vi "Configure Module.vi"(8 "error in (no error)":errorcluster, 10 "IOV ref in":refnum<k21>, 11 "9478 in":refnum<class "9478.lvclass">) -> (0 "error out":errorcluster, 2 "IOV ref out":refnum<k21>, 3 "9478 out":refnum<class "9478.lvclass">)   [LabVIEW 2019, in "Modules.lvlib" / "9478.lvclass"]
uses:
  9478.lvclass
  9478.lvclass/9478.ctl
  <resource>/objmgr/cRIO.rc
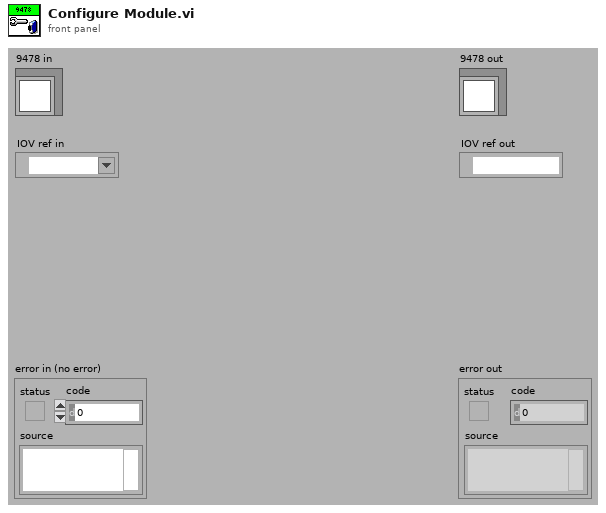
[diagram p1: front panel]
types:
  T1 = typedef "Modules.lvlib/9478.lvclass/Active Limit.ctl" = u8
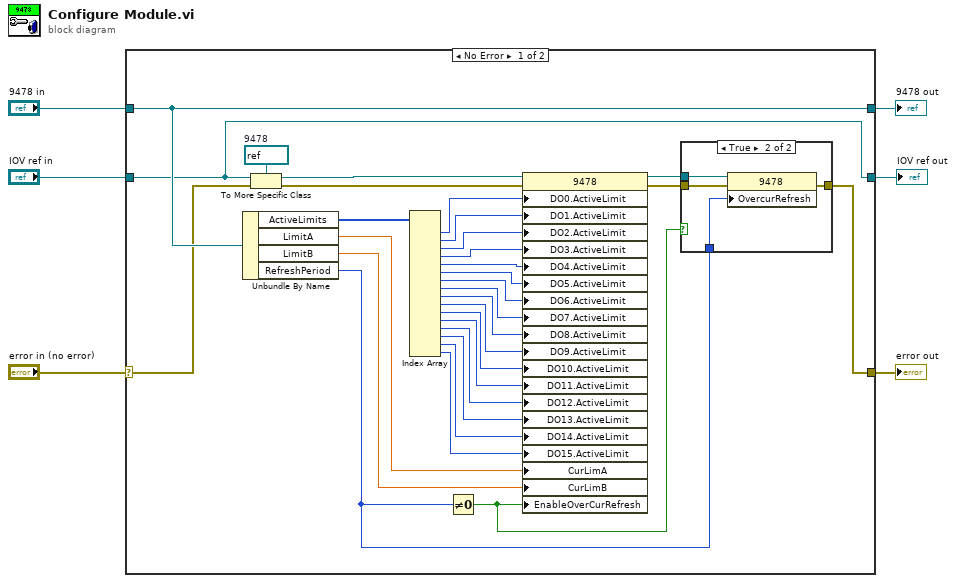
[diagram p0: block diagram]
diagram:
  n1 = case shown="No Error" "error in (no error)" {
    selector: "error in (no error)" -> [w35 w44]
    tunnel: [w9 w44] -> w5
    tunnel: [w36 w43] -> w3
    tunnel: "9478 in" -> [w36 w43]
    tunnel: "IOV ref in" -> [w31 w42]
    tunnel: [w31 w42] -> w1
    frame No Error {
      w34 = refnum<k21> refnum  # 9478
      n2 = Unbundle By Name(w36) -> ("ActiveLimits"=w30:T1[], "LimitA"=w13:dbl, "LimitB"=w12:dbl, "RefreshPeriod"=w7:u8)
      n3 = To More Specific Class(target class=w34, reference=w31, error in=w35) -> (specific class reference=w33:refnum<k21>, error out=w32:errorcluster)
      n4 = Index Array(array=w30) -> (element #1=w29:T1, element #2=w28:T1, element #3=w27:T1, element #4=w26:T1, element #5=w25:T1, element #6=w24:T1, element #7=w23:T1, element #8=w22:T1, element #9=w21:T1, element #10=w20:T1, element #11=w19:T1, element #12=w18:T1, element #13=w17:T1, element #14=w16:T1, element #15=w15:T1, element #16=w14:T1)  [unwired: 16 in]
      n5 = Not Equal To 0?(x=w7) -> (x != 0?=w8:bool)
      n6 = property class="9478"(reference=w33, error in=w32, "DO0.ActiveLimit"=w29, "DO1.ActiveLimit"=w28, "DO2.ActiveLimit"=w27, "DO3.ActiveLimit"=w26, "DO4.ActiveLimit"=w25, "DO5.ActiveLimit"=w24, "DO6.ActiveLimit"=w23, "DO7.ActiveLimit"=w22, "DO8.ActiveLimit"=w21, "DO9.ActiveLimit"=w20, "DO10.ActiveLimit"=w19, "DO11.ActiveLimit"=w18, "DO12.ActiveLimit"=w17, "DO13.ActiveLimit"=w16, "DO14.ActiveLimit"=w15, "DO15.ActiveLimit"=w14, "CurLimA"=w13, "CurLimB"=w12, "EnableOverCurRefresh"=w8) -> (reference out=w11:refnum<k21>, error out=w10:errorcluster)
      n7 = case shown="True" w8 {
        tunnel: w11 -> [_ w41]
        tunnel: w10 -> [w37 w40]
        tunnel: [w37 w39] -> w9
        tunnel: w7 -> [_ w38]
        frame False {
        }
        frame True {
          n8 = property class="9478"(reference=w41, error in=w40, "OvercurRefresh"=w38) -> (error out=w39:errorcluster)  [unwired: 1 out]
        }
      }
    }
    frame Error {
    }
  }
  "error out" <- w5
  "9478 out" <- w3
  "IOV ref out" <- w1
